vi "超限报警数组.vi"() -> ()   [LabVIEW 2012]
panel:
  out "超限报警数组":cluster{"数值 2":dbl, "颜色盒 2":u32}[][](array[cluster])
  out "数值":dbl
  out "颜色盒":u32(colorbox)
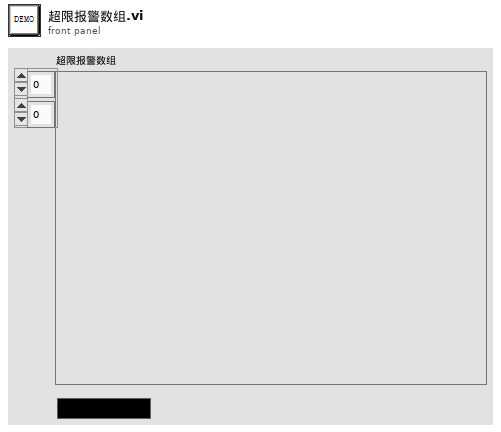
[diagram p1: front panel]
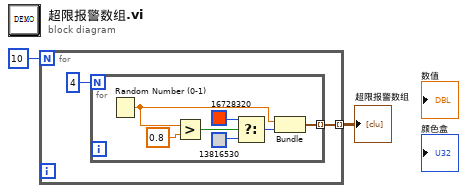
[diagram p0: block diagram]
diagram:
  n1 = for {
    N: 10 -> [_]
    tunnel: [w3] -> w1 mode=indexing
    n2 = for {
      N: 4 -> [_]
      tunnel: [w6] -> w3 mode=indexing
      n3 = Random Number (0-1)() -> (number: 0 to 1=w5:dbl)
      n4 = Greater?(x=w5, y=0.8) -> (0:w7:bool)
      n5 = Select(t=u32 16728320 ("颜色盒"), s=w7, f=u32 13816530 ("颜色盒")) -> (s? t:f=w8:u32)
      n6 = Bundle("number: 0 to 1"=w5, "颜色盒"=w8) -> (w6:cluster{"number: 0 to 1":dbl, "颜色盒":u32})  [unwired: 1 in]
    }
  }
  "超限报警数组" <- w1
